vi "Global 2.vi"() -> ()   [LabVIEW 2017]
panel:
  in  "Star Auto":bool
  in  "EMG":bool
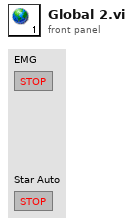
[diagram p1: front panel]
diagram:
